vi "Shooter Motor.vi"(6 "On/Off":bool, 8 "Shooter State Input":T1(ring), 9 "Motor Time (s)":dbl, 10 "Extend Time (s)":dbl, 11 "Trigger":bool) -> (0 "Shooter State Output":T1(ring), 2 "State":string, 3 "Ready":bool)   [LabVIEW 2012]
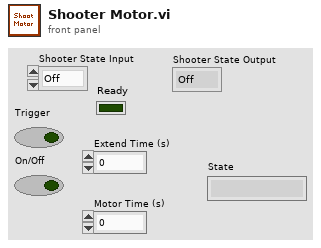
[diagram p1: front panel]
types:
  T1 = enum16{"Off", "Starting Initial", "Starting", "On"}
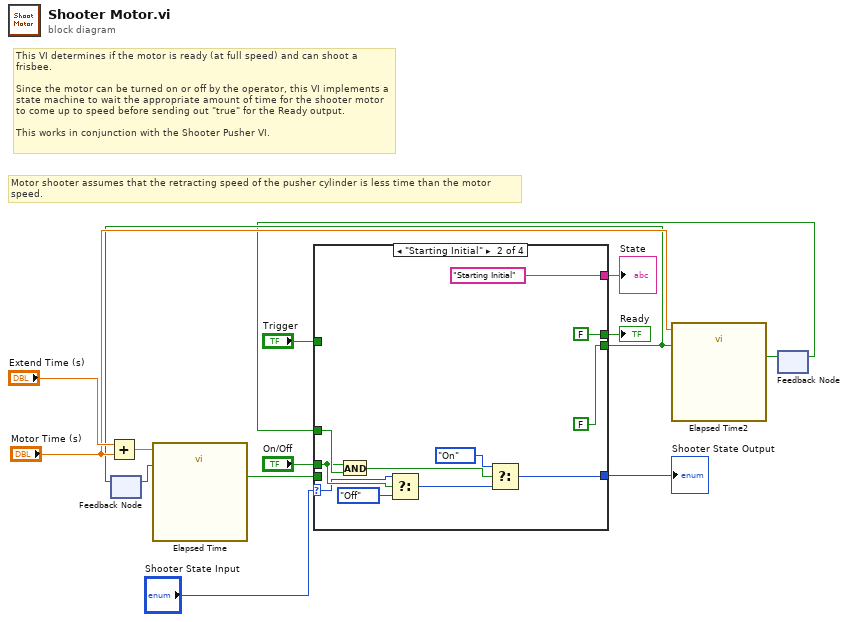
[diagram p0: block diagram]
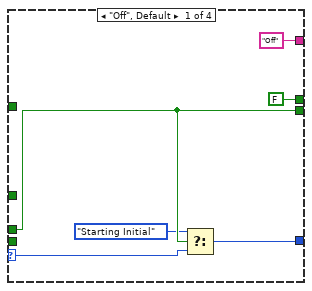
[diagram p2: hidden frame]
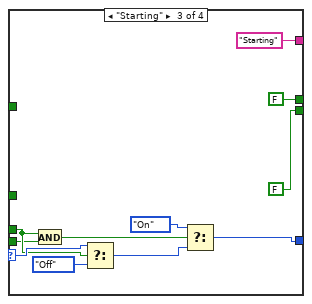
[diagram p3: hidden frame]
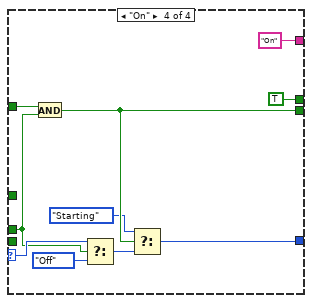
[diagram p4: hidden frame]
diagram:
  # "This VI determines if the motor is ready (at full speed) and can shoot a frisbee.\n\nSince the motor can be turned on or off by the operator, this VI implements a\nstate machine to wait the appropriate amount of time for the shooter motor\nto come up to speed before sending out \"true\" for the Ready output.\n\nThis works in conjunction with the Shooter Pusher VI."
  # "Motor shooter assumes that the retracting speed of the pusher cylinder is less time than the motor speed."
  n1 = Add(x="Extend Time (s)", y="Motor Time (s)") -> (x+y=w11:dbl)
  n2 = feedback #1() -> (w10:bool)  [unwired: 1 in]
  n3 = call "Elapsed Time"("Time Target (s)"=w11, "Reset"=w10) -> ("Time has Elapsed"=w13:bool)  [unwired: 10 in, 7 out]
  n4 = feedback #2() -> (w6:bool)  [unwired: 1 in]
  n5 = case shown="\"Starting Initial\"" "Shooter State Input" {
    selector: "Shooter State Input" -> [w20 w24 w38 w50]
    tunnel: "On/Off" -> [w17 w25 w37 w47]
    tunnel: [w16 w23 w42 w48] -> w2
    tunnel: [FALSE FALSE ("Ready") FALSE TRUE ("Ready")] -> w5
    tunnel: ["Off" "Starting Initial" "Starting" "On"] -> w14
    tunnel: [w17 FALSE ("On") FALSE ("On") w46] -> w8
    tunnel: w13 -> [_ _ w34 _]
    tunnel: w6 -> [_ w26 _ _]
    tunnel: "Trigger" -> [_ _ _ w43]
    frame "Off", Default {
      n6 = Select(t=T1."Starting Initial", s=w17, f=w20) -> (s? t:f=w16:T1)
    }
    frame "Starting Initial" {
      n7 = And(x=w25, y=w26) -> (x .and. y?=w30:bool)
      n8 = Select(t=w24, s=w25, f=T1."Off") -> (s? t:f=w29:T1)
      n9 = Select(t=T1."On", s=w30, f=w29) -> (s? t:f=w23:T1)
    }
    frame "Starting" {
      n10 = And(x=w37, y=w34) -> (x .and. y?=w36:bool)
      n11 = Select(t=w38, s=w37, f=T1."Off") -> (s? t:f=w35:T1)
      n12 = Select(t=T1."On", s=w36, f=w35) -> (s? t:f=w42:T1)
    }
    frame "On" {
      n13 = And(x=w43, y=w47) -> (x .and. y?=w46:bool)
      n14 = Select(t=w50, s=w47, f=T1."Off") -> (s? t:f=w49:T1)
      n15 = Select(t=T1."Starting", s=w46, f=w49) -> (s? t:f=w48:T1)
    }
  }
  "Shooter State Output" <- w2
  "Ready" <- w5
  "State" <- w14
  n16 = feedback-in #1(w8) -> ()
  n17 = call "Elapsed Time2"("Time Target (s)"="Motor Time (s)", "Reset"=w8) -> ("Time has Elapsed"=w7:bool)  [unwired: 10 in, 7 out]
  n18 = feedback-in #2(w7) -> ()
